vi "Hasdouble_value.vi"(8 "error in (no error)":errorcluster, 11 "OneOfTemplate in":refnum<class "ni_protobuf_types_WaveformAttributeValue_attribute.lvclass">) -> (0 "error out":errorcluster, 2 "Has Data?":bool, 3 "OneOfTemplate out":refnum<class "ni_protobuf_types_WaveformAttributeValue_attribute.lvclass">)   [LabVIEW 2020, in "ni.protobuf.types.lvlib" / "ni_protobuf_types_WaveformAttributeValue_attribute.lvclass"]
uses:
  ni_protobuf_types_WaveformAttributeValue_attribute.lvclass
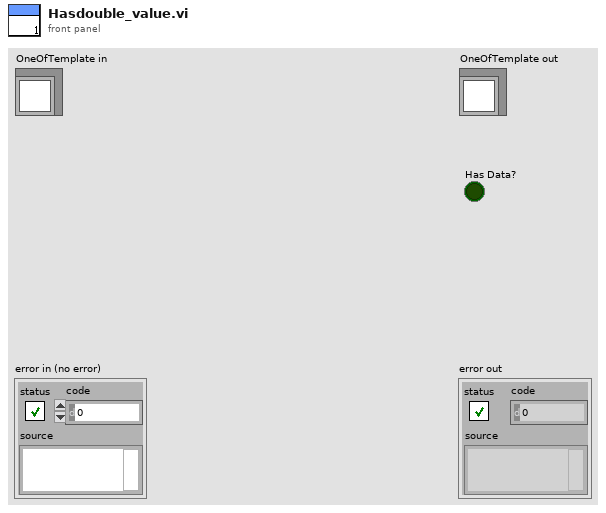
[diagram p1: front panel]
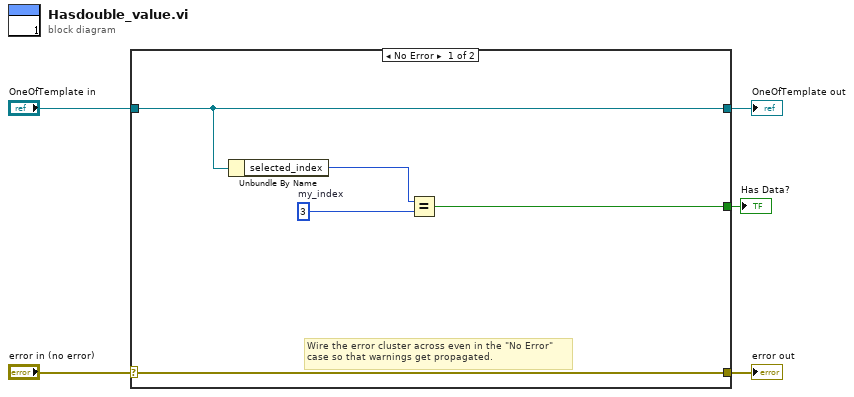
[diagram p0: block diagram]
diagram:
  n1 = case shown="No Error" "error in (no error)" {
    selector: "error in (no error)" -> [w10 w12]
    tunnel: [w10 w12] -> w4
    tunnel: [w9 w11] -> w2
    tunnel: "OneOfTemplate in" -> [w9 w11]
    tunnel: [w6 _] -> w1
    frame No Error {
      w7 = 3  # my_index
      # "Wire the error cluster across even in the \"No Error\"\ncase so that warnings get propagated."
      n2 = Unbundle By Name(w9) -> ("selected_index"=w8:i32)
      n3 = Equal?(x=w8, y=w7) -> (x = y?=w6:bool)
    }
    frame Error {
    }
  }
  "error out" <- w4
  "OneOfTemplate out" <- w2
  "Has Data?" <- w1
